vi "Polygon Intersection_Find Bottom.vi"(4 "index2":i32, 6 "index1":i32, 7 "Left Turn?":bool, 8 "y2":dbl[](array[numeric]), 9 "x2":dbl[](array[numeric]), 10 "y1":dbl[](array[numeric]), 11 "x1":dbl[](array[numeric])) -> (0 "y":dbl, 1 "x":dbl, 2 "index2 out":i32, 3 "index1 out":i32, 5 "isolate?":bool)   [LabVIEW 2020, in "NI_AAL_Geometry.lvlib"]
uses:
  <vilib>/Analysis/NI_AAL_Geometry.lvlib
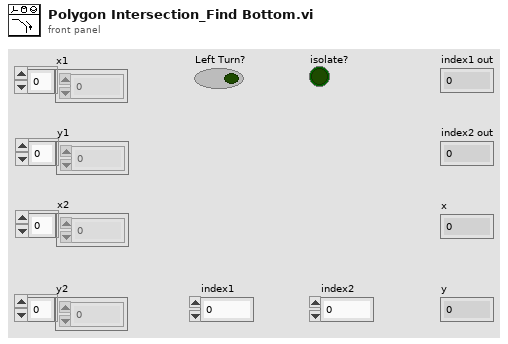
[diagram p1: front panel]
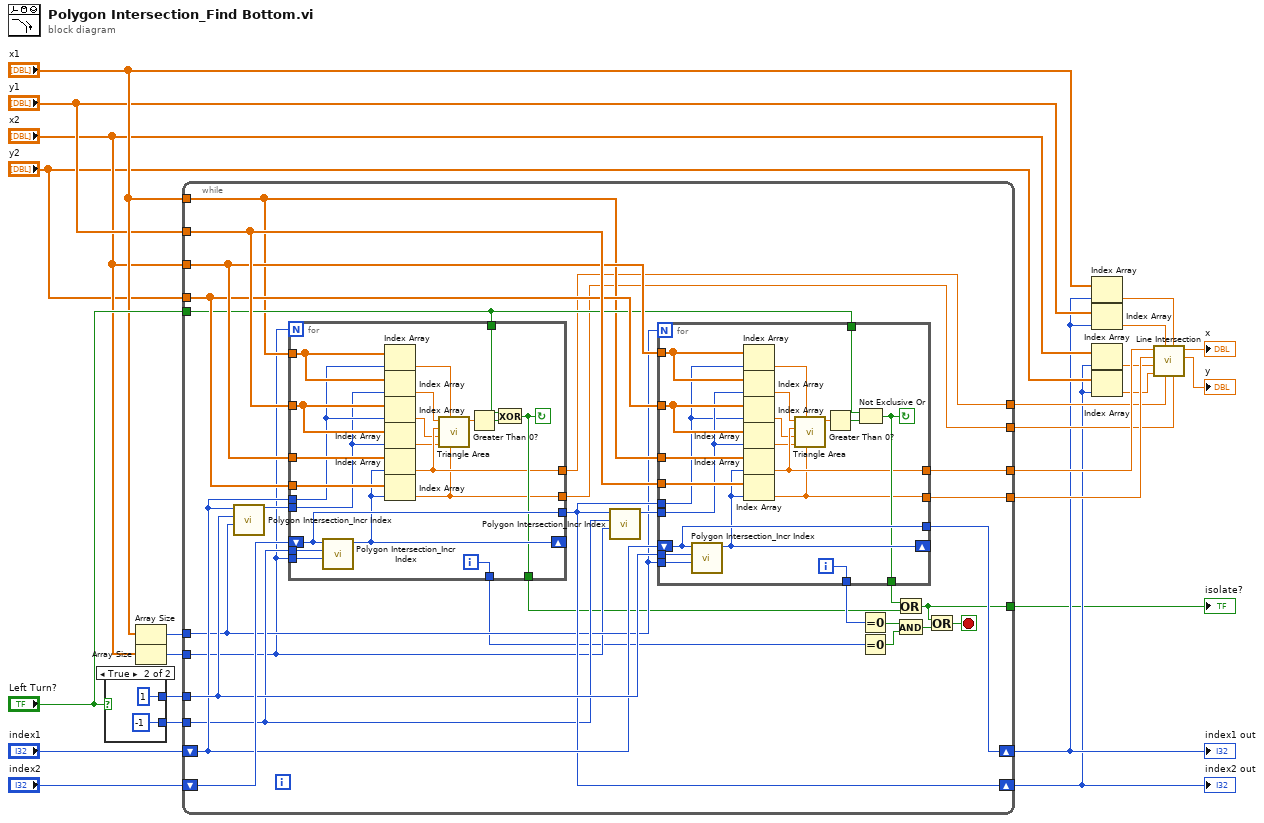
[diagram p0: block diagram]
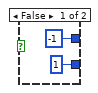
[diagram p2: hidden frame]
diagram:
  n1 = case shown="True" "Left Turn?" {
    tunnel: [-1 1] -> w23
    tunnel: [1 -1] -> w24
    frame False {
    }
    frame True {
    }
  }
  n2 = Array Size(array="x1") -> (size(s)=w2:i32)
  n3 = Array Size(array="x2") -> (size(s)=w1:i32)
  n4 = while {
    tunnel: "x1" -> [w49]
    tunnel: "y1" -> [w56]
    tunnel: "x2" -> [w55]
    tunnel: "y2" -> [w54]
    tunnel: w24 -> [w38]
    tunnel: w23 -> [w43]
    tunnel: w2 -> [w37]
    tunnel: w1 -> [w36]
    tunnel: "Left Turn?" -> [w50]
    tunnel: [w48] -> w11
    tunnel: [w47] -> w10
    tunnel: [w46] -> w7
    tunnel: [w45] -> w6
    shift-right: [w44] -> w5
    shift-left: "index1" -> [w41]
    shift-right: [w39] -> w4
    shift-left: "index2" -> [w53]
    tunnel: [w35] -> w3
    stop <- w29 stop-if-true
    n5 = call <vilib>:"Polygon Intersection_Incr Index.vi"("polygon size"=w37, "incr"=w43, "index"=w41) -> ("incr index"=w42:i32)  [unwired: 8 in]
    n6 = for {
      N: w36 -> [_]
      tunnel: w49 -> [w95]
      tunnel: w56 -> [w96]
      tunnel: w55 -> [w98]
      tunnel: w54 -> [w97]
      tunnel: w38 -> [w92]
      tunnel: w42 -> [w87]
      shift-right: [w91] -> _
      shift-left: w53 -> [w93]
      tunnel: [w93] -> w39
      tunnel: [w94] -> w33
      tunnel: w36 -> [w90]
      tunnel: w50 -> [w89]
      tunnel: [w83] -> w46
      tunnel: [w80] -> w45
      tunnel: w41 -> [w88]
      tunnel: [w86] -> w31
      i -> [w94]
      stop <- w86 continue-if-true
      n7 = call <vilib>:"Polygon Intersection_Incr Index.vi"("polygon size"=w90, "incr"=w92, "index"=w93) -> ("incr index"=w91:i32)  [unwired: 8 in]
      n8 = Index Array(array=w95, index=w88) -> (element=w85:dbl)
      n9 = Index Array(array=w95, index=w87) -> (element=w84:dbl)
      n10 = Index Array(array=w96, index=w88) -> (element=w82:dbl)
      n11 = Index Array(array=w96, index=w87) -> (element=w81:dbl)
      n12 = Index Array(array=w98, index=w91) -> (element=w83:dbl)
      n13 = Index Array(array=w97, index=w91) -> (element=w80:dbl)
      n14 = call <vilib>:"Triangle Area.vi"("y 3"=w80, "x 1"=w85, "y 2"=w81, "y 1"=w82, "x 3"=w83, "x 2"=w84) -> ("area"=w79:dbl)  [unwired: 5 in]
      n15 = Greater Than 0?(x=w79) -> (x > 0?=w78:bool)
      n16 = Exclusive Or(1:w78, 2:w89) -> (0:w86:bool)
    }
    n17 = call <vilib>:"Polygon Intersection_Incr Index.vi"("polygon size"=w36, "incr"=w38, "index"=w39) -> ("incr index"=w40:i32)  [unwired: 8 in]
    n18 = for {
      N: w37 -> [_]
      tunnel: w49 -> [w75]
      tunnel: w56 -> [w74]
      tunnel: w55 -> [w77]
      tunnel: w54 -> [w76]
      tunnel: w43 -> [w72]
      shift-right: [w70] -> _
      shift-left: w41 -> [w71]
      tunnel: [w71] -> w44
      tunnel: [w73] -> w34
      tunnel: w37 -> [w69]
      tunnel: w50 -> [w68]
      tunnel: [w62] -> w48
      tunnel: [w59] -> w47
      tunnel: w40 -> [w67]
      tunnel: w39 -> [w66]
      tunnel: [w65] -> w32
      i -> [w73]
      stop <- w65 continue-if-true
      n19 = call <vilib>:"Polygon Intersection_Incr Index.vi"("polygon size"=w69, "incr"=w72, "index"=w71) -> ("incr index"=w70:i32)  [unwired: 8 in]
      n20 = Index Array(array=w77, index=w66) -> (element=w64:dbl)
      n21 = Index Array(array=w77, index=w67) -> (element=w63:dbl)
      n22 = Index Array(array=w76, index=w66) -> (element=w61:dbl)
      n23 = Index Array(array=w76, index=w67) -> (element=w60:dbl)
      n24 = Index Array(array=w75, index=w70) -> (element=w62:dbl)
      n25 = Index Array(array=w74, index=w70) -> (element=w59:dbl)
      n26 = call <vilib>:"Triangle Area.vi"("y 3"=w59, "x 1"=w64, "y 2"=w60, "y 1"=w61, "x 3"=w62, "x 2"=w63) -> ("area"=w58:dbl)  [unwired: 5 in]
      n27 = Greater Than 0?(x=w58) -> (x > 0?=w57:bool)
      n28 = Not Exclusive Or(1:w57, 2:w68) -> (0:w65:bool)
    }
    n29 = Equal To 0?(x=w34) -> (x = 0?=w52:bool)
    n30 = Equal To 0?(x=w33) -> (x = 0?=w51:bool)
    n31 = Or(x=w32, y=w31) -> (x .or. y?=w35:bool)
    n32 = And(x=w52, y=w51) -> (x .and. y?=w30:bool)
    n33 = Or(x=w35, y=w30) -> (x .or. y?=w29:bool)
  }
  "index1 out" <- w5
  "index2 out" <- w4
  "isolate?" <- w3
  n34 = Index Array(array="x1", index=w5) -> (element=w15:dbl)
  n35 = Index Array(array="y1", index=w5) -> (element=w14:dbl)
  n36 = Index Array(array="x2", index=w4) -> (element=w9:dbl)
  n37 = Index Array(array="y2", index=w4) -> (element=w8:dbl)
  n38 = call <vilib>:"Line Intersection.vi"("y 4"=w6, "x 1"=w15, "x 4"=w7, "y 1"=w14, "y 3"=w8, "x 3"=w9, "y 2"=w10, "x 2"=w11) -> ("y"=→"y":dbl, "x"=→"x":dbl)  [unwired: 2 in]
